vi "Master Identifyer.vi"(8 "error in (no error) 2":errorcluster, 11 "VISA resource name":refnum<visa-resource-name>) -> (0 "error out (no error)":errorcluster, 1 "Class out":refnum<class "Universal Power Meter.lvclass">, 2 "ID cluster.Model":string, 3 "ID cluster.Manufacturer":string, 4 "THD?":bool)   [LabVIEW 2014, in "Universal Power Meter.lvlib" / "Universal Power Meter.lvclass"]
uses:
  Universal Power Meter.lvclass
  Generic Instrument/Generic Instrument.lvclass
panel:
  out "Option String":string
  out "ID":string
  out "Instrument ID":string
  out "Power Meter Visa":refnum<visa-resource-name>
  out "Number of Cards":dbl
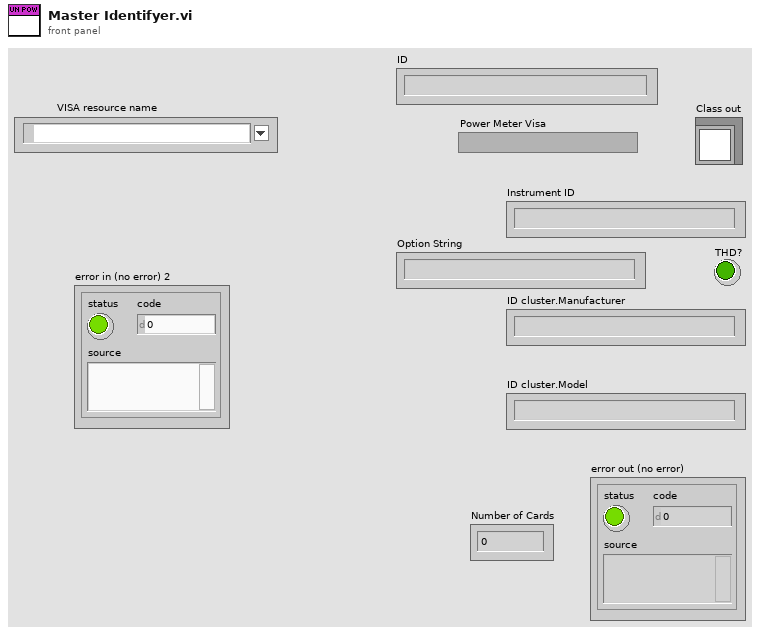
[diagram p1: front panel]
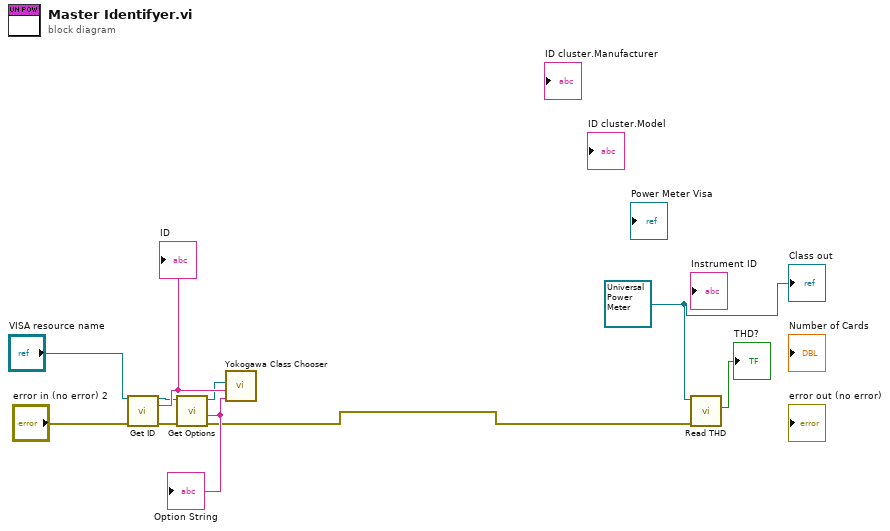
[diagram p0: block diagram]
diagram:
  w1 = refnum<class "Universal Power Meter.lvclass"> refnum ("Class out")
  n1 = call "Get ID.vi"("VISA resource name"="VISA resource name", "error in (no error)"="error in (no error) 2") -> ("VISA resource name 2"=w8:refnum<visa-resource-name>, "ID"=w9:string, "error out"=w5:errorcluster)  [unwired: 9 in, 2 out]
  "ID" <- w9
  n2 = call "Get Options.vi"("error in (no error)"=w5, "VISA resource name"=w8) -> ("error out"=w2:errorcluster, "Option String"=w6:string, "VISA resource name 2"=w7:refnum<visa-resource-name>)  [unwired: 7 in]
  "Option String" <- w6
  n3 = call "Yokogawa Class Chooser.vi"("Incoming Otpion"=w6, "Incoming ID"=w9, "VISA resource name"=w7) -> ()  [unwired: 8 in, 1 out]
  n4 = call-dynamic "Read THD.vi"("error in (no error)"=w2, "Universal Power Meter in"=w1) -> ("THD?"=→"THD?":bool)  [unwired: 7 in, 2 out]
  "Class out" <- w1
